vi "Find Common Chars.vi"(10 "Reference":string, 11 "Target":string) -> (3 "Common":string)   [LabVIEW 2020]
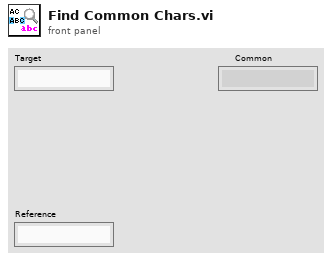
[diagram p1: front panel]
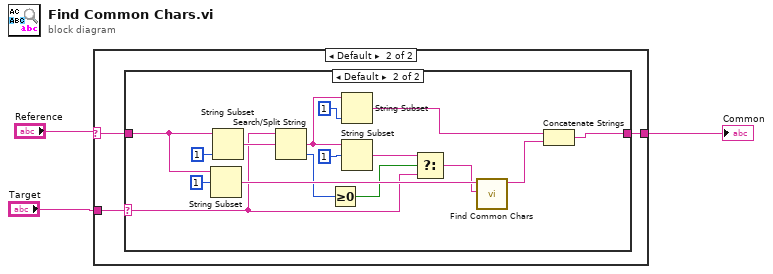
[diagram p0: block diagram]
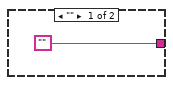
[diagram p2: hidden frame]
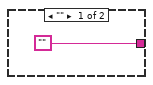
[diagram p3: hidden frame]
diagram:
  n1 = case shown="Default" "Reference" {
    selector: "Reference" -> [_ w7]
    tunnel: "Target" -> [_ w6]
    tunnel: ["" w5] -> w3
    frame "" {
    }
    frame Default {
      n2 = case shown="Default" w6 {
        selector: w6 -> [_ w10]
        tunnel: w7 -> [_ w22]
        tunnel: ["" w21] -> w5
        frame "" {
        }
        frame Default {
          n3 = String Subset(string=w22, offset (0)=1 ("length (rest)")) -> (substring=w19:string)  [unwired: 1 in]
          n4 = String Subset(string=w22, length (rest)=1 ("length (rest)")) -> (substring=w16:string)  [unwired: 1 in]
          n5 = Search/Split String(string=w10, search string/char (-)=w16) -> (match + rest of string=w13:string, offset of match=w9:i32)  [unwired: 1 in, 1 out]
          n6 = Greater Or Equal To 0?(x=w9) -> (x >= 0?=w18:bool)
          n7 = String Subset(string=w13, length (rest)=1 ("length (rest)")) -> (substring=w12:string)  [unwired: 1 in]
          n8 = String Subset(string=w13, offset (0)=1 ("length (rest)")) -> (substring=w11:string)  [unwired: 1 in]
          n9 = Select(t=w11, s=w18, f=w10) -> (s? t:f=w17:string)
          n10 = call "Find Common Chars.vi"("Reference"=w17, "Target"=w19) -> ("Common"=w20:string)  [unwired: 9 in]
          n11 = Concatenate Strings(w12, w20) -> (w21:string)
        }
      }
    }
  }
  "Common" <- w3
